vi "诊断标定3.vi"(8 "CAN端口":u16(ring), 9 "设备索引号":u16(ring), 10 "CAN卡类型":u32(ring)=21) -> ()   [LabVIEW 2013] (continued)
      n10 = property on="电池实际容量(A)" class="DigNum (严格)"("Disabled"=w43) -> ()  [unwired: 2 in, 2 out]
      n11 = property on="使用者" class="DigNum (严格)"("Disabled"=w43) -> ()  [unwired: 2 in, 2 out]
      n12 = property on="SOH(%)" class="DigNum (严格)"("Disabled"=w43) -> ()  [unwired: 2 in, 2 out]
      n13 = property on="电池额定容量(A)" class="DigNum (严格)"("Disabled"=w43) -> ()  [unwired: 2 in, 2 out]
      n14 = local write "主从选择"(enum32{"主板", "从板"}."主板" ("主从选择")) -> ()
      n15 = property on="SOC(%)" class="DigNum (严格)"("Disabled"=w43) -> ()  [unwired: 2 in, 2 out]
      n16 = local write "等级 2"(T19."从板信息" ("等级 2")) -> ()
      n17 = local write "主板2"(T8."项目信息" ("主从板")) -> ()
      n18 = property class="MCListbox (严格)"(reference=w48, "ItemNames"=w44) -> ()  [unwired: 1 in, 2 out]
      n19 = property class="MCListbox (严格)"(reference=w47, "ItemNames"=w44) -> ()  [unwired: 1 in, 2 out]
      n20 = property class="MCListbox (严格)"(reference=w46, "ItemNames"=w44) -> ()  [unwired: 1 in, 2 out]
      n21 = property class="Bool (严格)"(reference=w65, "BoolText.TextColor"=u32 87470) -> ()  [unwired: 1 in, 2 out]
      n22 = property class="Bool (严格)"(reference=w66, "BoolText.TextColor"=w40) -> ()  [unwired: 1 in, 2 out]
      n23 = local write "主从板"(enum32{"单选选项2", "单选选项1"}."单选选项1" ("主从板")) -> ()
      n24 = property on="项目信息2" class="Clust (严格)"("DisabledEnum"=w43) -> ()  [unwired: 2 in, 2 out]
      n25 = property on="系统时钟" class="Str"("Disabled"=w43) -> ()  [unwired: 2 in, 2 out]
      n26 = property on="配置文件版本" class="Str"("Disabled"=w43) -> ()  [unwired: 2 in, 2 out]
      n27 = property on="车架(牌)号" class="Str"("Disabled"=w43) -> ()  [unwired: 2 in, 2 out]
      n28 = property on="产品编号" class="Str"("Disabled"=w43) -> ()  [unwired: 2 in, 2 out]
      n29 = property on="从板号" class="DigNum (严格)"("NumText.BGColor"=w40) -> ()  [unwired: 2 in, 2 out]
      n30 = property on="单选选项2 2" class="Bool (严格)"("BoolText.TextColor"=w40) -> ()  [unwired: 2 in, 2 out]
      n31 = local write "面板选择"(T7."读写参数" ("面板选择")) -> ()
      n32 = property on="单选选项1" class="Bool (严格)"("BoolText.TextColor"=u32 5898201) -> ()  [unwired: 2 in, 2 out]
      n33 = property on="单选选项2" class="Bool (严格)"("BoolText.TextColor"=w40) -> ()  [unwired: 2 in, 2 out]
      n34 = local write "主界面选项"(enum32{"单选选项1", "单选选项2", "单选选项2 2", "单选选项2 3"}."单选选项1" ("主界面选项")) -> ()
      n35 = local write "判定3"(w50) -> ()
      n36 = local write "清BUFF"(w50) -> ()
      n37 = local write "1"(w50) -> ()
      n38 = property on="从板个数" class="DigNum (严格)"("Visible"=w50) -> ()  [unwired: 2 in, 2 out]
      n39 = property on="从板个数" class="DigNum (严格)"("NumText.BGColor"=u32 16448250) -> ()  [unwired: 2 in, 2 out]
      n40 = Not(x=w50) -> (.not. x?=w69:bool)
      n41 = local write "布尔"(w50) -> ()
      n42 = property on="主板选项" class="Tree (严格)"("Visible"=w50) -> ()  [unwired: 2 in, 2 out]
      n43 = property on="全部写入" class="Bool (严格)"("DisabledEnum"=2) -> ()  [unwired: 2 in, 2 out]
      n44 = property on="当前从板板号" class="DigNum (严格)"("Visible"=w69) -> ()  [unwired: 2 in, 2 out]
      n45 = property on="从板选项" class="Tree (严格)"("Visible"=w69) -> ()  [unwired: 2 in, 2 out]
      n46 = control-ref of="结果"() -> (w56:refnum<vi>)
      n47 = control-ref of="结果"() -> (w53:refnum<vi>)
      n48 = local write "强制停止版本读取"(w42) -> ()
      n49 = local write "强制终止读写标记"(w42) -> ()
      n50 = control-ref of="项目信息"() -> (w54:refnum<vi>)
      n51 = local write "判定2"(w42) -> ()
      n52 = local write "停止"(w42) -> ()
      n53 = local write "控制1"(w42) -> ()
      n54 = local write "消除"(w42) -> ()
      n55 = global write "EV05全局变量1.vi" "授权功能"(w42) -> ()
      n56 = local write "继电器超时处理"(w42) -> ()
      n57 = local write "1 6"(w42) -> ()
      n58 = local write "1 7"(w42) -> ()
      n59 = local write "1 8"(w42) -> ()
      n60 = local write "1 9"(w42) -> ()
      n61 = local write "1 10"(w42) -> ()
      n62 = local write "1 2"(w42) -> ()
      n63 = local write "1 3"(w42) -> ()
      n64 = local write "1 4"(w42) -> ()
      n65 = local write "1 5"(w42) -> ()
      n66 = local write "1 11"(w42) -> ()
      n67 = for {
        N: 100 -> [_]
        tunnel: w56 -> [w95]
        i -> [w93]
        n68 = Bundle(w93, 0) -> (w91:cluster{i32, i32})  [unwired: 1 out]
        n69 = property class="MCListbox (严格)"(reference=w95, "ActiveCell"=w91, "CellBG"=u32 16448250) -> ()  [unwired: 1 in, 2 out]
      }
      n70 = for {
        N: 100 -> [_]
        tunnel: w54 -> [w90]
        i -> [w89]
        n71 = Bundle(w89, 0) -> (w87:cluster{i32, i32})  [unwired: 1 out]
        n72 = property class="Tbl (严格)"(reference=w90, "Active Cell"=w87, "Cell BG Color"=u32 16448250) -> ()  [unwired: 1 in, 2 out]
      }
      n73 = for {
        N: 100 -> [_]
        tunnel: w53 -> [w100]
        i -> [w98]
        n74 = Bundle(w98, 0) -> (w96:cluster{i32, i32})  [unwired: 1 out]
        n75 = property class="MCListbox (严格)"(reference=w100, "ActiveCell"=w96, "CellBG"=u32 16448250) -> ()  [unwired: 1 in, 2 out]
      }
      n76 = stacked-sequence {
        tunnel: [_ w74] -> w49
        frame #0 {
          n77 = local read "设备索引号"() -> (w71:u16)
          n78 = local read "CAN卡类型"() -> (w70:u32)
          n79 = local read "CAN端口"() -> (w72:u16)
          n80 = dll-call lib="PTH1tabs FBluewave New EnergySVN_Work\nBNET01_BMStrunkBMS_Monitor_增加二维码data\nkerneldlls\nusbcan.dll" fn="VCI_ClearBuffer"("DeviceType"=w70, "DeviceInd"=w71, "CANInd"=w72) -> (error out=w73:errorcluster)  [unwired: 4 in, 4 out]
          n81 = call <vilib>:"Clear Errors.vi"("error in (no error)"=w73) -> ()  [unwired: 6 in, 1 out]
        }
        frame #1 {
          w81 = u8 0 items=["Normal", "Listen Only"] ("工作方式")
          w80 = u8 1 items=["Dual Filter", "Single Filter"] ("滤波方式")
          n82 = local read "设备索引号"() -> (w76:u16)
          n83 = local read "CAN卡类型"() -> (w75:u32)
          n84 = local read "CAN端口"() -> (w77:u16)
          n85 = call "CAN_Init-8.6.vi"("CAN卡类型"=w75, "设备索引号"=w76, "CAN端口"=w77, "操作类型"=enum16{"初始化CAN", "关闭CAN"}."初始化CAN", "滤波方式"=w80, "Accept Code"=u32 3221225472, "簇"=T21 {"打开CAN"=FALSE, "初始化CAN"=TRUE, "开始CAN"=TRUE, "重启"=FALSE, "关闭CAN"=FALSE}, "Mask Code"=u32 1073741823 ("Accept Code"), "工作方式"=w81, "是否滤波"=TRUE, "滤波选择"=T20 {"fiter_mode"=1, "fiter_endid"=402653184, "fiter_startid"=419430399}) -> ("error out"=w74:errorcluster)  [unwired: 3 in, 5 out]
        }
      }
      n86 = local write "加热继电器(从)"(w42) -> ()
      n87 = local write "风机继电器(从)"(w42) -> ()
      n88 = local write "DO1"(w42) -> ()
      n89 = local write "DO2"(w42) -> ()
      n90 = local write "DO1 2"(w42) -> ()
      n91 = local write "正级继电器"(w42) -> ()
      n92 = local write "负级继电器"(w42) -> ()
      n93 = local write "加热继电器"(w42) -> ()
      n94 = local write "充电继电器"(w42) -> ()
      n95 = local write "风机继电器"(w42) -> ()
      n96 = local write "预充电继电器"(w42) -> ()
      n97 = property on="保存版本信息" class="Bool (严格)"("Visible"=w42) -> ()  [unwired: 2 in, 2 out]
      n98 = property on="单个读取" class="Bool (严格)"("Visible"=w42) -> ()  [unwired: 2 in, 2 out]
      n99 = property on="单个写入" class="Bool (严格)"("Visible"=w42) -> ()  [unwired: 2 in, 2 out]
      n100 = local write "正级继电器 12"(w42) -> ()
      n101 = local write "正级继电器 2"(w42) -> ()
      n102 = local write "正级继电器 3"(w42) -> ()
      n103 = local write "正级继电器 4"(w42) -> ()
      n104 = local write "正级继电器 5"(w42) -> ()
      n105 = local write "正级继电器 6"(w42) -> ()
      n106 = local write "正级继电器 7"(w42) -> ()
      n107 = local write "正级继电器 8"(w42) -> ()
      n108 = local write "正级继电器 9"(w42) -> ()
      n109 = local write "正级继电器 10"(w42) -> ()
      n110 = local write "正级继电器 11"(w42) -> ()
      n111 = property on="从板号" class="DigNum (严格)"("Visible"=w42) -> ()  [unwired: 2 in, 2 out]
      "电池故障" <- w44
      "模块版本值" <- w61
      "硬件版本" <- w62
      "模块版本名称" <- w61
      "平台软件版本" <- w62
      "项目软件版本" <- w62
      "模块个数" <- u8[] [0, 0, 0, 0, 0, 0, 0, 0, 0, 0, 0, 0, 0, 0, 0, 0, 0, 0, 0, 0, 0, 0, 0, 0, 0, 0, 0, 0, 0, 0, 0, 0] ("模块个数")
    }
  }
  n112 = stacked-sequence {
    tunnel: [w101] -> w23
    frame #0 {
      n113 = call <vilib>:"Set Busy.vi"() -> ()  [unwired: 10 in, 2 out]
      n114 = disable-structure shown="禁用" {
        frame Disabled {
          n115 = control-ref of="主板选项"() -> (w220:refnum<vi>)
          n116 = stacked-sequence {
            tunnel: w220 -> [w222 w380 w418]
            frame #0 {
              # "加热和充电控制参数"
              n117 = global read "功能码全局.vi" "主板控制类信息10"() -> (w232:bool[])
              n118 = Index Array(array=w232) -> (element #5=w226:bool, element #6=w224:bool, element #7=w225:bool, element #8=w223:bool)  [unwired: 8 in, 4 out]
              n119 = Not Or(1:w225, 2:w226) -> (0:w231:bool)
              n120 = Not Or(1:w223, 2:w224) -> (0:w229:bool)
              n121 = for {
                N: 8 -> [_]
                tunnel: w222 -> [w352]
                tunnel: w231 -> [w348]
                tunnel: [w347] -> w230
                i -> [w350]
                n122 = Add(x=w350, y=69) -> (x+y=w351:i32)
                n123 = property class="Tree (严格)"(reference=w352, "Active Item Row Number"=w351, "Disabled?"=w348) -> (error out=w347:errorcluster)  [unwired: 1 in, 1 out]
              }
              n124 = for {
                N: 9 -> [_]
                tunnel: w222 -> [w346]
                tunnel: w229 -> [w342]
                tunnel: w230 -> [w341]
                tunnel: [w340] -> w221
                i -> [w344]
                n125 = Add(x=w344, y=77) -> (x+y=w345:i32)
                n126 = property class="Tree (严格)"(reference=w346, error in=w341, "Active Item Row Number"=w345, "Disabled?"=w342) -> (error out=w340:errorcluster)  [unwired: 1 out]
              }
              n127 = stacked-sequence {
                tunnel: w222 -> [w252 _ _]
                tunnel: w221 -> [w251 _ _]
                frame #0 {
                  # "电池信息"
                  n128 = global read "功能码全局.vi" "主板版本号11"() -> (w253:bool[])
                  n129 = global read "功能码全局.vi" "主板项目信息4"() -> (w235:bool[])
                  n130 = Index Array(array=w253) -> (element #1=w249:bool, element #2=w248:bool, element #3=w242:bool, element #4=w236:bool, element #6=w241:bool, element #7=w240:bool, element #8=w239:bool)  [unwired: 8 in, 1 out]
                  n131 = Index Array(array=w235, index=4 ("索引")) -> (element=w233:bool)
                  n132 = Or(x=w242, y=w236) -> (x .or. y?=w237:bool)
                  n133 = Not(x=w240) -> (.not. x?=w244:bool)
                  n134 = Not(x=w239) -> (.not. x?=w243:bool)
                  n135 = Not(x=w241) -> (.not. x?=w245:bool)
                  n136 = property on="硬件版本号" class="Str"("Visible"=w242) -> ()  [unwired: 2 in, 2 out]
                  n137 = property on="读硬件版本号" class="Bool (严格)"("Visible"=w242) -> ()  [unwired: 2 in, 2 out]
                  n138 = property on="项目软件版本号" class="Str"("Visible"=w242) -> ()  [unwired: 2 in, 2 out]
                  n139 = property on="项目软本读取" class="Bool (严格)"("Visible"=w242) -> ()  [unwired: 2 in, 2 out]
                  n140 = property on="继电器屏1 2" class="TabCtl (严格)"("Visible"=w245) -> ()  [unwired: 2 in, 2 out]
                  n141 = property on="均衡屏" class="TabCtl (严格)"("Visible"=w243) -> ()  [unwired: 2 in, 2 out]
                  n142 = property on="继电器屏1 2" class="TabCtl (严格)"("Visible"=w245) -> ()  [unwired: 2 in, 2 out]
                  n143 = property on="DO屏" class="TabCtl (严格)"("Visible"=w244) -> ()  [unwired: 2 in, 2 out]
                  n144 = Compound Arithmetic op=OR(w241, w240, w239) -> (w238:bool)
                  n145 = Not Or(1:w248, 2:w249) -> (0:w247:bool)
                  n146 = stacked-sequence {
                    tunnel: w238 -> [_ w258 _]
                    tunnel: w237 -> [_ _ w262]
                    tunnel: w233 -> [w254 _ _]
                    frame #0 {
                      n147 = case shown="真" w254 {
                        frame False {
                        }
                        frame True {
                          n148 = local write "主界面选项"(enum32{"单选选项1", "单选选项2", "单选选项2 2", "单选选项2 3"}."单选选项2 3" ("主界面选项")) -> ()
                          n149 = local write "面板选择"(T7."高压板校正" ("面板选择")) -> ()
                        }
                      }
                      n150 = control-ref of="单选选项2 3"() -> (w255:refnum<vi>)
                      n151 = property class="Bool (严格)"(reference=w255, "Visible"=w254) -> ()  [unwired: 1 in, 2 out]
                    }
                    frame #1 {
                      n152 = control-ref of="单选选项2 2"() -> (w259:refnum<vi>)
                      n153 = case shown="真" w258 {
                        frame False {
                        }
                        frame True {
                          n154 = local write "主界面选项"(enum32{"单选选项1", "单选选项2", "单选选项2 2", "单选选项2 3"}."单选选项2 2" ("主界面选项")) -> ()
                          n155 = local write "面板选择"(enum32{"读写参数", "版本读取", "其它诊断"}."其它诊断" ("选项卡控件 2")) -> ()
                        }
                      }
                      n156 = property class="Bool (严格)"(reference=w259, "Visible"=w258) -> ()  [unwired: 1 in, 2 out]
                    }
                    frame #2 {
                      n157 = control-ref of="单选选项2"() -> (w263:refnum<vi>)
                      n158 = case shown="真" w262 {
                        frame False {
                        }
                        frame True {
                          n159 = local write "主界面选项"(enum32{"单选选项1", "单选选项2", "单选选项2 2", "单选选项2 3"}."单选选项2" ("主界面选项")) -> ()
                          n160 = local write "面板选择"(enum32{"读写参数", "版本读取", "其它诊断"}."版本读取" ("选项卡控件 2")) -> ()
                        }
                      }
                      n161 = property class="Bool (严格)"(reference=w263, "Visible"=w262) -> ()  [unwired: 1 in, 2 out]
                    }
                  }
                  n162 = for {
                    N: 5 -> [_]
                    tunnel: w252 -> [w272]
                    tunnel: w247 -> [w268]
                    tunnel: w251 -> [w267]
                    tunnel: [w266] -> w250
                    i -> [w270]
                    n163 = Add(x=w270, y=86) -> (x+y=w271:i32)
                    n164 = property class="Tree (严格)"(reference=w272, error in=w267, "Active Item Row Number"=w271, "Disabled?"=w268) -> (error out=w266:errorcluster)  [unwired: 1 out]
                  }
                  n165 = property on="模块软件版本 2" class="MCListbox (严格)"("Visible"=w236) -> ()  [unwired: 2 in, 2 out]
                  n166 = property on="模块软件版本" class="Enum (严格)"("Visible"=w236) -> ()  [unwired: 2 in, 2 out]
                  n167 = property on="平台软件版本号" class="Str"("Visible"=w236) -> ()  [unwired: 2 in, 2 out]
                  n168 = property on="模块版本读取" class="Bool (严格)"("Visible"=w236) -> ()  [unwired: 2 in, 2 out]
                  n169 = property on="平台软件版本读取" class="Bool (严格)"("Visible"=w236) -> ()  [unwired: 2 in, 2 out]
                  n170 = call <vilib>:"Clear Errors.vi"("error in (no error)"=w250) -> ()  [unwired: 6 in, 1 out]
                }
                frame #1 {
                  n171 = global read "功能码全局.vi" "主板项目信息7"() -> (w312:bool[])
                  n172 = global read "功能码全局.vi" "主板控制类信息10"() -> (w308:bool[])
                  n173 = global read "功能码全局.vi" "主板故障阀值9"() -> (w311:bool[])
                  n174 = global read "功能码全局.vi" "主板项目信息4"() -> (w290:bool[])
                  n175 = global read "功能码全局.vi" "主板项目信息5"() -> (w299:bool[])
                  n176 = global read "功能码全局.vi" "主板项目信息6"() -> (w289:bool[])
                  n177 = global read "功能码全局.vi" "主板版本号11"() -> (w298:bool[])
                  n178 = Delete From Array(array=w289, length=1 ("长度"), index=0 ("索引")) -> (deleted portion=w300:bool[], array with subset deleted=w316:bool[])
                  n179 = Index Array(array=w290, index #1=5 ("索引"), index #2=6 ("索引"), index #3=7 ("索引")) -> (element #1=w301:bool, element #2=w317:bool, element #3=w273:bool)
                  n180 = Index Array(array=w298) -> (element #1=w305:bool, element #2=w321:bool)  [unwired: 2 in]
                  n181 = Array Subset(array=w311, index=2 ("索引"), length=3 ("长度")) -> (w303:bool[])
                  n182 = Delete From Array(array=w312, length=3 ("索引"), index=2 ("长度")) -> (deleted portion=w302:bool[], array with subset deleted=w318:bool[])
                  n183 = Array Subset(array=w308, index=4 ("索引"), length=2 ("长度")) -> (w304:bool[])
                  n184 = global read "功能码全局.vi" "18"() -> (w281:bool[])
                  n185 = global read "功能码全局.vi" "16"() -> (w282:bool[])
                  n186 = Insert Into Array(array=w299, new element #1=w300, new element #2=w301, new element #3=w302, new element #4=w303, new element #5=w304, new element #6=w305) -> (w322:bool[])  [unwired: 1 in]
                  n187 = Array Subset(array=w308, index=6 ("索引"), length=2 ("长度")) -> (w320:bool[])
                  n188 = Array Subset(array=w311, index=5 ("索引"), length=3 ("长度")) -> (w319:bool[])
                  n189 = And Array Elements(Boolean array=w322) -> (logical AND=w287:bool)
                  n190 = Array Subset(array=w281, index=0 ("索引"), length=8 ("长度")) -> (w279:bool[])
                  n191 = Array Subset(array=w282, index=4 ("索引"), length=4 ("长度")) -> (w278:bool[])
                  n192 = Or Array Elements(Boolean array=w322) -> (logical OR=w274:bool)
                  n193 = Insert Into Array(array=w316, new element #1=w317, new element #2=w318, new element #3=w319, new element #4=w320, new element #5=w321) -> (w323:bool[])  [unwired: 1 in]
                  n194 = property on="全部读取" class="Bool (严格)"("Visible"=w287) -> ()  [unwired: 2 in, 2 out]
                  n195 = global read "功能码全局.vi" "15"() -> (w280:bool[])
                  n196 = And Array Elements(Boolean array=w323) -> (logical AND=w288:bool)
                  n197 = property on="全部写入" class="Bool (严格)"("Visible"=w288) -> ()  [unwired: 2 in, 2 out]
                  n198 = Or Array Elements(Boolean array=w323) -> (logical OR=w324:bool)
                  n199 = Insert Into Array(array=w280, new element #1=w279, new element #2=w278) -> (w277:bool[])  [unwired: 1 in]
                  n200 = Or Array Elements(Boolean array=w277) -> (logical OR=w276:bool)
                  n201 = Compound Arithmetic op=OR(w273, w274, w324, w276) -> (w325:bool)
                  n202 = case shown="真" w325 {
                    frame False {
                    }
                    frame True {
                      n203 = local write "主界面选项"(enum32{"单选选项1", "单选选项2", "单选选项2 2", "单选选项2 3"}."单选选项1" ("主界面选项")) -> ()
                      n204 = local write "面板选择"(enum32{"读写参数", "版本读取", "其它诊断"}."读写参数" ("选项卡控件 2")) -> ()
                    }
                  }
                  n205 = property on="单选选项1" class="Bool (严格)"("Visible"=w325) -> ()  [unwired: 2 in, 2 out]
                }
                frame #2 {
                  n206 = control-ref of="单选选项2 2"() -> (w332:refnum<vi>)
                  n207 = control-ref of="单选选项2 3"() -> (w328:refnum<vi>)
                  n208 = control-ref of="单选选项2"() -> (w334:refnum<vi>)
                  n209 = control-ref of="单选选项1"() -> (w333:refnum<vi>)
                  n210 = local read "主界面选项"() -> (w337:enum32{"单选选项1", "单选选项2", "单选选项2 2", "单选选项2 3"})
                  n211 = Build Array(w333, w334, w332, w328) -> (w331:refnum<vi>[])
                  n212 = Delete From Array(array=w331, index=w337) -> (deleted portion=w335:refnum<vi>, array with subset deleted=w336:refnum<vi>[])  [unwired: 1 in]
                  n213 = property class="Bool (严格)"(reference=w335, "BoolText.TextColor"=u32 87470) -> ()  [unwired: 1 in, 2 out]
                  n214 = for {
                    tunnel: u32 16777215 -> [w339]
                    tunnel: w336 -> [w338] mode=indexing
                    n215 = property class="Bool (严格)"(reference=w338, "BoolText.TextColor"=w339) -> ()  [unwired: 1 in, 2 out]
                  }
                }
              }
            }
            frame #1 {
              # "项目信息"
              # "SOC"
              # "SOH"
              # "电池额定实际容量"
              # "车牌号"
              # "产品编号"
              # "电压个数"
              # "通道电压数"
              # "温度个数"
              # "电压起始值"
              # "温度起始值"
              # "配置文件版本"
              # "系统时钟"
              # "校正时钟"
              n216 = global read "功能码全局.vi" "主板项目信息5"() -> (w413:bool[])
              n217 = global read "功能码全局.vi" "主板项目信息6"() -> (w412:bool[])
              n218 = global read "功能码全局.vi" "主板项目信息7"() -> (w389:bool[])
              n219 = global read "功能码全局.vi" "主板项目信息4"() -> (w360:bool[])
              n220 = Index Array(array=w413) -> (element #1=w410:bool, element #2=w407:bool, element #3=w404:bool, element #4=w401:bool, element #5=w397:bool, element #6=w395:bool, element #7=w392:bool, element #8=w388:bool)  [unwired: 8 in]
              n221 = Index Array(array=w412) -> (element #1=w385:bool, element #2=w409:bool, element #3=w406:bool, element #4=w403:bool, element #5=w400:bool, element #6=w396:bool, element #7=w394:bool, element #8=w391:bool)  [unwired: 8 in]
              n222 = Index Array(array=w389) -> (element #1=w387:bool, element #2=w384:bool, element #3=w382:bool, element #4=w377:bool, element #5=w374:bool, element #6=w381:bool, element #7=w375:bool, element #8=w373:bool)  [unwired: 8 in]
              n223 = Index Array(array=w360) -> (element #6=w356:bool, element #7=w355:bool, element #8=w359:bool)  [unwired: 8 in, 5 out]
              n224 = Not(x=w359) -> (.not. x?=w358:bool)
              n225 = Not Or(1:w355, 2:w356) -> (0:w354:bool)
              n226 = Not Or(1:w409, 2:w410) -> (0:w372:bool)
              n227 = Not Or(1:w406, 2:w407) -> (0:w371:bool)
              n228 = Not Or(1:w403, 2:w404) -> (0:w370:bool)
              n229 = Not Or(1:w400, 2:w401) -> (0:w369:bool)
              n230 = Not Or(1:w396, 2:w397) -> (0:w368:bool)
              n231 = Not Or(1:w394, 2:w395) -> (0:w367:bool)
              n232 = Not Or(1:w391, 2:w392) -> (0:w366:bool)
              n233 = Not Or(1:w387, 2:w388) -> (0:w365:bool)
              n234 = Not Or(1:w381, 2:w382) -> (0:w363:bool)
              n235 = Not Or(1:w373, 2:w374) -> (0:w361:bool)
              n236 = Not Or(1:w375, 2:w377) -> (0:w362:bool)
              n237 = Not Or(1:w384, 2:w385) -> (0:w364:bool)
              n238 = Compound Arithmetic op=OR(w358, w372, w371, w370, w369, w368, w367, w366, w365, w364, w363, w362, w361) -> (w353:bool)
              "项目信息结果" <- w353
              n239 = property class="Tree (严格)"(reference=w380, "Active Item Row Number"=9 ("活动项:行数"), "Disabled?"=w354, "Active Item Row Number"=1 ("活动项:行数"), "Disabled?"=w353, "Active Item Row Number"=0 ("活动项:行数"), "Disabled?"=w358, "Active Item Row Number"=3 ("活动项:行数"), "Disabled?"=w372, "Active Item Row Number"=4 ("活动项:行数"), "Disabled?"=w371, "Active Item Row Number"=5 ("活动项:行数"), "Disabled?"=w370, "Active Item Row Number"=6 ("活动项:行数"), "Disabled?"=w369, "Active Item Row Number"=7 ("活动项:行数"), "Disabled?"=w368, "Active Item Row Number"=8 ("活动项:行数"), "Disabled?"=w367, "Active Item Row Number"=11 ("活动项:行数"), "Disabled?"=w366, "Active Item Row Number"=12 ("活动项:行数"), "Disabled?"=w365, "Active Item Row Number"=13 ("活动项:行数"), "Disabled?"=w364, "Active Item Row Number"=2 ("活动项:行数"), "Disabled?"=w363, "Active Item Row Number"=10 ("活动项:行数"), "Disabled?"=w362, "Active Item Row Number"=14 ("活动项:行数"), "Disabled?"=w361) -> ()  [unwired: 1 in, 2 out]
            }
            frame #2 {
              w423 = 18
              # "一二三级故障"
              n240 = global read "功能码全局.vi" "主板故障阀值9"() -> (w429:bool[])
              n241 = Index Array(array=w429) -> (element #3=w428:bool, element #4=w425:bool, element #5=w422:bool, element #6=w427:bool, element #7=w424:bool, element #8=w421:bool)  [unwired: 8 in, 2 out]
              n242 = Not Or(1:w427, 2:w428) -> (0:w417:bool)
              n243 = Not Or(1:w424, 2:w425) -> (0:w415:bool)
              n244 = Not Or(1:w421, 2:w422) -> (0:w416:bool)
              n245 = for {
                N: w423 -> [_]
                tunnel: w418 -> [w449]
                tunnel: w417 -> [w445]
                tunnel: [w444] -> w426
                i -> [w447]
                n246 = Add(x=w447, y=15) -> (x+y=w448:i32)
                n247 = property class="Tree (严格)"(reference=w449, "Active Item Row Number"=w448, "Disabled?"=w445) -> (error out=w444:errorcluster)  [unwired: 1 in, 1 out]
              }
              n248 = for {
                N: w423 -> [_]
                tunnel: w418 -> [w443]
                tunnel: w415 -> [w439]
                tunnel: w426 -> [w438]
                tunnel: [w437] -> w420
                i -> [w441]
                n249 = Add(x=w441, y=33) -> (x+y=w442:i32)
                n250 = property class="Tree (严格)"(reference=w443, error in=w438, "Active Item Row Number"=w442, "Disabled?"=w439) -> (error out=w437:errorcluster)  [unwired: 1 out]
              }
              n251 = for {
                N: w423 -> [_]
                tunnel: w418 -> [w436]
                tunnel: w416 -> [w432]
                tunnel: w420 -> [w431]
                tunnel: [w430] -> w419
                i -> [w434]
                n252 = Add(x=w434, y=51) -> (x+y=w435:i32)
                n253 = property class="Tree (严格)"(reference=w436, error in=w431, "Active Item Row Number"=w435, "Disabled?"=w432) -> (error out=w430:errorcluster)  [unwired: 1 out]
              }
              n254 = call <vilib>:"Clear Errors.vi"("error in (no error)"=w419) -> ()  [unwired: 6 in, 1 out]
            }
          }
        }
        frame Enabled {
        }
      }
      n255 = disable-structure shown="禁用" {
        disable-tunnel: [w102 _] -> w101
        frame Disabled {
          n256 = control-ref of="从板选项"() -> (w103:refnum<vi>)
          n257 = stacked-sequence {
            tunnel: w103 -> [w106 w143 w185]
            tunnel: [w104 _ _] -> w102
            frame #0 {
              n258 = global read "功能码全局.vi" "15"() -> (w129:bool[])
              n259 = global read "功能码全局.vi" "16"() -> (w120:bool[])
              n260 = Index Array(array=w129) -> (element #1=w128:bool, element #2=w126:bool, element #3=w124:bool, element #4=w122:bool, element #5=w127:bool, element #6=w125:bool, element #7=w123:bool, element #8=w121:bool)  [unwired: 8 in]
              n261 = Index Array(array=w120) -> (element #5=w111:bool, element #6=w119:bool, element #7=w110:bool, element #8=w118:bool)  [unwired: 8 in, 4 out]
              n262 = Not Or(1:w118, 2:w119) -> (0:w108:bool)
              n263 = Not Or(1:w110, 2:w111) -> (0:w109:bool)
              n264 = Not Or(1:w127, 2:w128) -> (0:w114:bool)
              n265 = Not Or(1:w125, 2:w126) -> (0:w115:bool)
              n266 = Not Or(1:w123, 2:w124) -> (0:w116:bool)
              n267 = Not Or(1:w121, 2:w122) -> (0:w117:bool)
              n268 = Compound Arithmetic op=OR(w114, w115, w116, w117, w108) -> (w113:bool)
              "从板项目信息" <- w113
              n269 = property class="Tree (严格)"(reference=w106, "Active Item Row Number"=1 ("活动项:行数"), "Disabled?"=w113, "Active Item Row Number"=2 ("活动项:行数"), "Disabled?"=w114, "Active Item Row Number"=3 ("活动项:行数"), "Disabled?"=w115, "Active Item Row Number"=4 ("活动项:行数"), "Disabled?"=w116, "Active Item Row Number"=5 ("活动项:行数"), "Disabled?"=w117, "Active Item Row Number"=0 ("活动项:行数"), "Disabled?"=w109) -> (error out=w105:errorcluster)  [unwired: 1 in, 1 out]
              n270 = for {
                N: 8 -> [_]
                tunnel: w106 -> [w141]
                tunnel: w108 -> [w137]
                tunnel: w105 -> [w136]
                tunnel: [w135] -> w104
                i -> [w139]
                n271 = Add(x=w139, y=6) -> (x+y=w140:i32)
                n272 = property class="Tree (严格)"(reference=w141, error in=w136, "Active Item Row Number"=w140, "Disabled?"=w137) -> (error out=w135:errorcluster)  [unwired: 1 out]
              }
              n273 = call <vilib>:"Clear Errors.vi"("error in (no error)"=w104) -> ()  [unwired: 6 in, 1 out]
            }
            frame #1 {
              w154 = 8
              n274 = global read "功能码全局.vi" "18"() -> (w163:bool[])
              n275 = Index Array(array=w163) -> (element #1=w146:bool, element #2=w147:bool, element #3=w162:bool, element #4=w157:bool, element #5=w151:bool, element #6=w161:bool, element #7=w156:bool, element #8=w150:bool)  [unwired: 8 in]
              n276 = Not Or(1:w147, 2:w146) -> (0:w142:bool)
              n277 = property class="Tree (严格)"(reference=w143, "Active Item Row Number"=46 ("活动项:行数"), "Disabled?"=w142, "Active Item Row Number"=47 ("活动项:行数"), "Disabled?"=w142, "Active Item Row Number"=48 ("活动项:行数"), "Disabled?"=w142) -> ()  [unwired: 1 in, 2 out]
              n278 = Not Or(1:w150, 2:w151) -> (0:w149:bool)
              n279 = Not Or(1:w161, 2:w162) -> (0:w160:bool)
              n280 = Not Or(1:w156, 2:w157) -> (0:w155:bool)
              n281 = for {
                N: w154 -> [_]
                tunnel: w143 -> [w184]
                tunnel: w160 -> [w180]
                tunnel: "error out" -> [w179]
                tunnel: [w178] -> w158
                i -> [w182]
                n282 = Add(x=w182, y=14) -> (x+y=w183:i32)
                n283 = property class="Tree (严格)"(reference=w184, error in=w179, "Active Item Row Number"=w183, "Disabled?"=w180) -> (error out=w178:errorcluster)  [unwired: 1 out]
              }
              n284 = for {
                N: w154 -> [_]
                tunnel: w143 -> [w177]
                tunnel: w155 -> [w173]
                tunnel: w158 -> [w172]
                tunnel: [w171] -> w153
                i -> [w175]
                n285 = Add(x=w175, y=22) -> (x+y=w176:i32)
                n286 = property class="Tree (严格)"(reference=w177, error in=w172, "Active Item Row Number"=w176, "Disabled?"=w173) -> (error out=w171:errorcluster)  [unwired: 1 out]
              }
              n287 = for {
                N: w154 -> [_]
                tunnel: w143 -> [w170]
                tunnel: w149 -> [w166]
                tunnel: w153 -> [w165]
                tunnel: [w164] -> w152
                i -> [w168]
                n288 = Add(x=w168, y=30) -> (x+y=w169:i32)
                n289 = property class="Tree (严格)"(reference=w170, error in=w165, "Active Item Row Number"=w169, "Disabled?"=w166) -> (error out=w164:errorcluster)  [unwired: 1 out]
              }
              n290 = call <vilib>:"Clear Errors.vi"("error in (no error)"=w152) -> ()  [unwired: 6 in, 1 out]
            }
            frame #2 {
              n291 = global read "功能码全局.vi" "23"() -> (w209:bool[])
              n292 = global read "功能码全局.vi" "24"() -> (w207:bool[])
              n293 = Index Array(array=w209) -> (element #3=w208:bool, element #4=w205:bool, element #5=w203:bool, element #6=w201:bool, element #7=w199:bool, element #8=w197:bool)  [unwired: 8 in, 2 out]
              n294 = Index Array(array=w207) -> (element #3=w206:bool, element #4=w204:bool, element #5=w202:bool, element #6=w200:bool, element #7=w198:bool, element #8=w196:bool)  [unwired: 8 in, 2 out]
              n295 = Not Or(1:w206, 2:w208) -> (0:w195:bool)
              n296 = Not Or(1:w204, 2:w205) -> (0:w190:bool)
              n297 = Not Or(1:w202, 2:w203) -> (0:w191:bool)
              n298 = Not Or(1:w200, 2:w201) -> (0:w192:bool)
              n299 = Not Or(1:w198, 2:w199) -> (0:w194:bool)
              n300 = Not Or(1:w196, 2:w197) -> (0:w193:bool)
              n301 = Build Array(w195, w195, w194, w193, w192, w191, w190) -> (w188:bool[])
              n302 = And Array Elements(Boolean array=w188) -> (logical AND=w189:bool)
              n303 = Insert Into Array(array=w188, index=0 ("索引"), new element=w189) -> (w186:bool[])
              n304 = for {
                N: 8 -> [_]
                tunnel: w185 -> [w219]
                tunnel: w186 -> [w215] mode=indexing
                tunnel: errorcluster {"status"=FALSE, "code"=0, "source"=""} ("error out 2") -> [w214]
                tunnel: [w213] -> w211
                i -> [w217]
                n305 = Add(x=w217, y=38) -> (x+y=w218:i32)
                n306 = property class="Tree (严格)"(reference=w219, error in=w214, "Active Item Row Number"=w218, "Disabled?"=w215) -> (error out=w213:errorcluster)  [unwired: 1 out]
              }
              n307 = call <vilib>:"Clear Errors.vi"("error in (no error)"=w211) -> ()  [unwired: 6 in, 1 out]
            }
          }
        }
        frame Enabled {
        }
      }
    }
  }
  n308 = local write "项目信息 2"(string[][] [["电压个数", "36"], ["温度个数", "45"], ["第一个保险通道", "0"], ["第一个保险位置", "0"], ["第二个保险通道", "0"], ["第二个保险位置", "0"], ["第三个保险通道", "0"], ["第三个保险位置", "0"], ["第四个保险通道", "0"], ["第四个保险位置", "0"], ["第五个保险通道", "0"], ["第五个保险位置", "0"], ["第六个保险通道", "0"], ["第六个保险位置", "0"], ["第七个保险通道", "0"], ["第七个保险位置", "0"], ["第八个保险通道", "0"], ["第八个保险位置", "0"], ["第九个保险通道", "0"], ["第九个保险位置", "0"], ["第十个保险通道", "0"], ["第十个保险位置", "0"], ["第1通道电压个数", "11"], ["第2通道电压个数", "12"], ["第3通道电压个数", "12"], ["第4通道电压个数", "12"], ["第5通道电压个数", "12"]] ("项目信息 2")) -> ()
  n309 = Index Array(array=w13, index (col)=0 ("索引 (行)")) -> (element=w16:string[])  [unwired: 1 in]
  n310 = Index Array(array=w13, index (col)=1 ("禁用的索引 (列)")) -> (element=w6:string[])  [unwired: 1 in]
  n311 = local read "从板个数"() -> (w8:dbl)
  n312 = Array Subset(array=w16, index=0 ("索引"), length=w8) -> (w15:string[])
  n313 = Array Subset(array=w16, index=10 ("索引"), length=w8) -> (w14:string[])
  n314 = Array Subset(array=w6, index=0 ("索引"), length=w8) -> (w12:string[])
  n315 = Array Subset(array=w6, index=10 ("索引"), length=w8) -> (w7:string[])
  n316 = Insert Into Array(array=w15, new element=w14) -> (w5:string[])  [unwired: 1 in]
  n317 = Insert Into Array(array=w12, new element=w7) -> (w4:string[])  [unwired: 1 in]
  n318 = stacked-sequence {
    tunnel: w20 -> [_]
    tunnel: w23 -> [_]
    frame #0 {
      n319 = call <vilib>:"Unset Busy.vi"() -> ()  [unwired: 11 in, 1 out]
    }
  }
  n320 = Build Array(w5, w4) -> (w3:string[][])
  n321 = local write "停止"(FALSE ("停止")) -> ()
  n322 = Transpose 2D Array(2D array=w3) -> (transposed array=w2:string[][])
  n323 = Obtain Queue(name (unnamed)=w37, element data type=w37, error in (no error)=w20) -> (queue out=w36:refnum<queue>, error out=w35:errorcluster)  [unwired: 2 in, 1 out]
  n324 = local write "项目信息"(w2) -> ()
  n325 = Obtain Queue(element data type="读参数") -> (queue out=w25:refnum<queue>, error out=w24:errorcluster)  [unwired: 4 in, 1 out]
  n326 = while {
    tunnel: w25 -> [w461]
    tunnel: w24 -> [w460]
    tunnel: [w459] -> w28
    tunnel: [w458] -> w27
    tunnel: w20 -> [_]
    tunnel: w23 -> [w450]
    stop <- w457 stop-if-true
    n327 = local read "停止"() -> (w457:bool)
    n328 = local read "设备索引号"() -> (w454:u16)
    n329 = local read "CAN卡类型"() -> (w455:u32)
    n330 = local read "CAN端口"() -> (w453:u16)
    n331 = call "receiver-8.6.vi"("错误输入（无错误）"=w450, "CAN端口"=w453, "设备索引号"=w454, "CAN卡类型"=w455) -> ("错误输出"=w456:errorcluster, "输出簇"=w452:T22, "接收成功"=w451:bool)  [unwired: 3 out]
    n332 = call <vilib>:"Clear Errors.vi"("error in (no error)"=w456) -> ()  [unwired: 6 in, 1 out]
    n333 = case shown="真" w451 {
      tunnel: w460 -> [w462 w468]
      tunnel: w452 -> [_ w467]
      tunnel: w461 -> [w463 w466]
      tunnel: [w463 w465] -> w459
      tunnel: [w462 w464] -> w458
      frame False {
      }
      frame True {
        n334 = Enqueue Element(queue=w466, element=w467, error in (no error)=w468) -> (queue out=w465:refnum<queue>, error out=w464:errorcluster)  [unwired: 2 out]
      }
    }
  }
  n335 = while {
    tunnel: w25 -> [w476]
    tunnel: w24 -> [w475]
    stop <- w469 stop-if-true
    n336 = local read "停止"() -> (w469:bool)
    n337 = local read "控制1"() -> (w471:bool)
    n338 = Dequeue Element(queue=w476, timeout in ms (-1)=200 ("超时毫秒(-1)"), error in (no error)=w475) -> (element=w474:T3, error out=w473:errorcluster)  [unwired: 2 out]
    n339 = case shown="无错误" w473 {
      tunnel: w474 -> [w481 _]
      tunnel: "写?" -> [w478 _]
      tunnel: w471 -> [w477 _]
      frame No Error {
        n340 = Unbundle(w481) -> ("return type"=w480:u32, "pReceive"=w479:T23)
        n341 = for {
          N: w480 -> [_]
          tunnel: w479 -> [w485] mode=indexing
          tunnel: w478 -> [w483]
          tunnel: w477 -> [w482]
          n342 = Unbundle By Name(w485) -> ("ID"=w486:u32)
          n343 = call "ID解析.vi"("ID"=w486) -> ("PDU(1)"=w484:i32)  [unwired: 10 out]
          n344 = case shown="18" w484 {
            tunnel: w485 -> [_ w496]
            tunnel: w483 -> [_ w488]
            tunnel: w482 -> [_ w487]
            frame 0, Default {
            }
            frame 24 {
              n345 = local read "主从选择"() -> (w489:enum32{"主板", "从板"})
              n346 = local read "设备索引号"() -> (w492:u16)
              n347 = local read "CAN卡类型"() -> (w491:u32)
              n348 = local read "CAN端口"() -> (w493:u16)
              n349 = disable-structure shown="禁用" {
                disable-tunnel: w496 -> [w499 _]
                frame Disabled {
                  n350 = call "标定授权读取.vi"("VCI_Receive"=w499) -> ()  [unwired: 1 out]
                }
                frame Enabled {
                }
              }
              n351 = case shown="\"从板\"" w489 {
                tunnel: [0 ("FUNC") w498] -> w490
                frame "主板", Default {
                }
                frame "从板" {
                  n352 = local read "从板号"() -> (w498:u8)
                }
              }
              n353 = local read "面板选择"() -> (w495:T7)
              n354 = case shown="\"读写参数\", 默认" w495 {
                tunnel: w488 -> [w504 _ _ _]
                tunnel: "命令" -> [w505 w608 w863 w1003]
                tunnel: w489 -> [w514 _ w871 w1011]
                tunnel: w496 -> [_ _ _ _]
                tunnel: w496 -> [w510 w609 w865 w1005]
                tunnel: w493 -> [w509 w610 w866 w1006]
                tunnel: w492 -> [w508 w611 w867 w1007]
                tunnel: w491 -> [w507 w612 w868 w1008]
                tunnel: w490 -> [w506 _ w864 w1004]
                tunnel: w487 -> [w500 _ _ _]
                frame "读写参数", Default {
                  n355 = local read "命令序号"() -> (w503:u8)
                  n356 = call "多帧接收机制(EV05).vi"("can卡类型"=w507, "设备索引号"=w508, "CAN端口"=w509, "VCI_Receive"=w510, "命令"=w505, "板号"=w506, "写?"=w504, "命令序号"=w503) -> ("错误信号"=w501:bool, "错误代码"=w513:i32, "输出数组"=w512:u8[], "读错误代码"=w502:u8[], "结束信号"=w511:bool)  [unwired: 7 out]
                  n357 = case shown="假" w504 {
                    tunnel: w511 -> [w524 w591]
                    tunnel: w513 -> [w523 w590]
                    tunnel: w503 -> [w522 _]
                    tunnel: w512 -> [w521 _]
                    tunnel: w505 -> [w520 _]
                    tunnel: w514 -> [w518 w589]
                    tunnel: w502 -> [w517 _]
                    tunnel: w501 -> [w516 _]
                    tunnel: w500 -> [w515 _]
                    frame False {
                      # "读参数"
                      n358 = And(x=w515, y=w524) -> (x .and. y?=w519:bool)
                      n359 = case shown="真" w519 {
                        tunnel: w523 -> [_ w535]
                        tunnel: w522 -> [_ w534]
                        tunnel: w521 -> [_ w533]
                        tunnel: w520 -> [_ w532]
                        tunnel: w518 -> [_ w528]
                        tunnel: w517 -> [_ w526]
                        tunnel: w516 -> [_ w527]
                        frame False {
                        }
                        frame True {
                          n360 = case shown="假" w527 {
                            tunnel: w535 -> [w546 _]
                            tunnel: w534 -> [w545 _]
                            tunnel: w533 -> [w544 _]
                            tunnel: w532 -> [w542 _]
                            tunnel: w528 -> [w538 _]
                            tunnel: w526 -> [_ w574]
                            frame False {
                              n361 = case shown="\"主板\", 默认" w538 {
                                tunnel: [w548 _] -> w541
                                tunnel: [_ w562] -> w540
                                tunnel: [w547 _] -> w537
                                frame "主板", Default {
                                n362 = stacked-sequence {
                                tunnel: [_ w561] -> w548
                                tunnel: [w549 _] -> w547
                                frame #0 {
                                n363 = control-ref of="一级故障"() -> (w555:refnum<vi>)
                                n364 = control-ref of="一级故障 2"() -> (w557:refnum<vi>)
                                n365 = control-ref of="一级故障 3"() -> (w558:refnum<vi>)
                                n366 = control-ref of="加热控制参数"() -> (w559:refnum<vi>)
                                n367 = control-ref of="充电控制参数"() -> (w560:refnum<vi>)
                                n368 = control-ref of="电池信息"() -> (w553:refnum<vi>)
                                n369 = control-ref of="项目信息"() -> (w556:refnum<vi>)
                                n370 = control-ref of="项目信息2"() -> (w554:refnum<vi>)
                                n371 = control-ref of="高压参数"() -> (w552:refnum<vi>)
                                n372 = local read "主板数据"() -> (w551:T4)
                                n373 = Bundle(cluster=w551, "项目信息"=w556, "一级故障 4"=w554, "一级故障"=w555, "一级故障 2"=w557, "一级故障 3"=w558, "加热控制参数"=w559, "充电控制参数"=w560, "高压参数"=w552, "电池信息"=w553) -> (w550:T4)
                                n374 = control-ref of="二维码信息"() -> (w549:refnum<vi>)
                                n375 = local write "主板数据"(w550) -> ()
                                }
                                frame #1 {
                                n376 = control-ref of="主板数据"() -> (w561:refnum<vi>)
                                }
                                }
                                }
                                frame "从板" {
                                n377 = stacked-sequence {
                                tunnel: [_ w573] -> w562
                                frame #0 {
                                n378 = control-ref of="从板号"() -> (w567:refnum<vi>)
                                n379 = control-ref of="项目信息 2"() -> (w568:refnum<vi>)
                                n380 = control-ref of="电池组信息"() -> (w566:refnum<vi>)
                                n381 = control-ref of="加热控制参数"() -> (w569:refnum<vi>)
                                n382 = control-ref of="一级故障(从板)"() -> (w570:refnum<vi>)
                                n383 = control-ref of="二级故障(从板)"() -> (w571:refnum<vi>)
                                n384 = control-ref of="三级故障(从板)"() -> (w572:refnum<vi>)
                                n385 = control-ref of="均衡参数"() -> (w565:refnum<vi>)
                                n386 = local read "从板信息"() -> (w564:T2)
                                n387 = Bundle(cluster=w564, "从板号"=w567, "项目信息 2"=w568, "加热控制参数"=w569, "一级故障(从板)"=w570, "二级故障(从板)"=w571, "三级故障(从板)"=w572, "电池组信息(从板)"=w566, "均衡参数"=w565) -> (w563:T2)
                                n388 = local write "从板信息"(w563) -> ()
                                }
                                frame #1 {
                                n389 = control-ref of="从板信息"() -> (w573:refnum<vi>)
                                }
                                }
                                }
                              }
                              n390 = control-ref of="二维码信息 2"() -> (w536:refnum<vi>)
                              n391 = control-ref of="结果"() -> (w543:refnum<vi>)
                              n392 = control-ref of="从板个数"() -> (w539:refnum<vi>)
                              n393 = call "输出数据解析.vi"("主板引用"=w541, "从板引用"=w540, "板选择"=w538, "二维码信息"=w537, "错误代码"=w546, "命令序号"=w545, "输入数组"=w544, "命令"=w542, "进度引用"=w543, "从板个数"=w539, "从板二维码信息"=w536) -> ()  [unwired: 5 out]
                            }
                            frame True {
                              n394 = Index Array(array=w574, index #1=0 ("索引"), index #2=1 ("索引")) -> (element #1=w577:u8, element #2=w578:u8)
                              n395 = Join Numbers(hi=w577, lo=w578) -> ((hi.lo)=w576:u16)
                              n396 = Number To Hexadecimal String(2:w576) -> (0:w575:string)  [unwired: 1 out]
                              n397 = control-ref of="结果"() -> (w583:refnum<vi>)
                              n398 = Concatenate Strings("0x" ("字符串"), w575) -> (w584:string)
                              n399 = Build Array(w584) -> (w585:string[])
                              n400 = call "表格编辑.vi"("新元素/子数组"=w585, "活动单元格:单元格背景色"=u32 16740749, "MCListbox引用句柄"=w583) -> ()  [unwired: 9 out]
                            }
                          }
                          n401 = global write "EV05全局变量1.vi" "流控帧 2"(FALSE ("流控帧 2")) -> ()
                          n402 = global write "EV05全局变量1.vi" "输出数组"(i32[] []) -> ()
                          n403 = local write "控制1"(FALSE ("控制1")) -> ()
                          n404 = local write "消除"(FALSE ("消除")) -> ()
                        }
                      }
                    }
                    frame True {
                      # "写参数判定"
                      n405 = And(x="控制1", y=w591) -> (x .and. y?=w588:bool)
                      n406 = case shown="真" w588 {
                        tunnel: w590 -> [_ w598]
                        tunnel: w589 -> [_ w595]
                        frame False {
                        }
                        frame True {
                          n407 = call <vilib>:"Unset Busy.vi"() -> ()  [unwired: 2 in, 10 out]
                          n408 = case shown="\"主板\", 默认" w595 {
                            tunnel: [w599 w600] -> w597
                            frame "主板", Default {
                              n409 = local read "主板选项"() -> (w599:string)
                            }
                            frame "从板" {
                              n410 = local read "从板选项"() -> (w600:string)
                            }
                          }
                          n411 = control-ref of="结果"() -> (w596:refnum<vi>)
                          n412 = call "输入数据判定.vi"("主从选择"=w595, "主板选项"=w597, "进度引用"=w596, "错误代码"=w598) -> ()  [unwired: 2 in, 6 out]
                          n413 = global write "EV05全局变量1.vi" "流控帧 2"(FALSE ("流控帧 2")) -> ()
                          n414 = local write "控制1"(FALSE ("控制1")) -> ()
                          n415 = local write "消除"(FALSE ("消除")) -> ()
                        }
                      }
                      n416 = global write "EV05全局变量1.vi" "输出数组"(i32[] []) -> ()
                    }
                  }
                }
                frame "版本读取" {
                  n417 = local read "命令序号"() -> (w601:u8)
                  n418 = local read "从板板号"() -> (w604:u8)
                  n419 = local read "控制1"() -> (w605:bool)
                  n420 = call "多帧接收机制(EV05).vi"("can卡类型"=w612, "设备索引号"=w611, "CAN端口"=w610, "VCI_Receive"=w609, "命令"=w608, "板号"=w604, "命令序号"=w601) -> ("错误信号"=w602:bool, "输出数组"=w613:u8[], "读错误代码"=w603:u8[], "结束信号"=w607:bool)  [unwired: 1 in, 8 out]
                  n421 = And(x=w605, y=w607) -> (x .and. y?=w606:bool)
                  n422 = case shown="真" w606 {
                    tunnel: w613 -> [_ w621]
                    tunnel: w601 -> [_ w620]
                    tunnel: w608 -> [_ w619]
                    tunnel: w603 -> [_ w615]
                    tunnel: w602 -> [_ w614]
                    frame False {
                    }
                    frame True {
                      n423 = case shown="假" w614 {
                        tunnel: w621 -> [w625 _]
                        tunnel: w620 -> [w624 _]
                        tunnel: w619 -> [w623 _]
                        tunnel: w615 -> [w622 w849]
                        frame False {
                          n424 = case shown="89" w623 {
                            tunnel: w624 -> [_ w628]
                            tunnel: w625 -> [_ w627]
                            tunnel: w622 -> [_ _]
                            frame 0, Default {
                            }
                            frame 137 {
                              n425 = case shown="1" w628 {
                                tunnel: w627 -> [_ w656 w700 w720 w847]
                                frame 0, Default {
                                }
                                frame 1 {
                                w638 = "." ("字符串")
                                n426 = Array Subset(array=w656, index=0 ("索引"), length=14 ("长度")) -> (w669:u8[])
                                n427 = Index Array(array=w656, index=14 ("索引")) -> (element=w659:u8)
                                n428 = Index Array(array=w656, index #1=15 ("索引"), index #2=16 ("索引")) -> (element #1=w665:u8, element #2=w666:u8)
                                n429 = Index Array(array=w656, index #1=17 ("索引"), index #2=18 ("索引")) -> (element #1=w660:u8, element #2=w661:u8)
                                n430 = call "数组去零.vi"("输入"=w669) -> ("输出"=w644:dbl[])
                                n431 = Join Numbers(hi=w660, lo=w661) -> ((hi.lo)=w657:u16)
                                n432 = Join Numbers(hi=w665, lo=w666) -> ((hi.lo)=w658:u16)
                                n433 = Number To Decimal String(number=w659) -> (decimal integer string=w651:string)  [unwired: 1 out]
                                n434 = Byte Array To String(unsigned byte array=w644) -> (string=w643:string)
                                n435 = Number To Decimal String(number=w657) -> (decimal integer string=w639:string)  [unwired: 1 out]
                                n436 = Number To Decimal String(number=w658) -> (decimal integer string=w650:string)  [unwired: 1 out]
                                n437 = Array Subset(array=w656, index=21 ("索引"), length=7 ("长度")) -> (w653:u8[])
                                n438 = Concatenate Strings("V" ("字符串"), w651, w638, w650, w638, w639) -> (w648:string)
                                n439 = call "数组去零.vi"("输入"=w653) -> ("输出"=w636:dbl[])
                                n440 = Byte Array To String(unsigned byte array=w636) -> (string=w634:string)
                                n441 = call <vilib>:"Space Constant.vi"() -> ("String"=w635:string)
                                n442 = Equal?(x=w634, y=w635) -> (x = y?=w640:bool)
                                n443 = Concatenate Strings("-" ("字符串"), w634) -> (w641:string)
                                n444 = Select(t=w635, s=w640, f=w641) -> (s? t:f=w637:string)
                                n445 = Concatenate Strings(w643, "-" ("字符串"), w648, w637) -> (w630:string)
                                n446 = local read "项目软件版本"() -> (w632:string[])
                                n447 = local read "从板板号"() -> (w629:u8)
                                n448 = local write "项目软件版本号"(w630) -> ()
                                n449 = Replace Array Subset(array=w632, new element=w630, index=w629) -> (w631:string[])
                                n450 = control-ref of="结果"() -> (w647:refnum<vi>)
                                n451 = local write "项目软件版本"(w631) -> ()
                                n452 = Build Array("项目软件版本     读取完成" ("读取结果")) -> (w645:string[])
                                n453 = call "表格编辑(版本读取).vi"("新元素/子数组"=w645, "活动单元格:单元格背景色"=u32 6618880, "MCListbox引用句柄"=w647) -> ()  [unwired: 9 out]
                                }
                                frame 2 {
                                w683 = ""
                                w680 = "." ("字符串")
                                n454 = Array Subset(array=w700, index=0 ("索引"), length=14 ("长度")) -> (w688:u8[])
                                n455 = Index Array(array=w700, index=14 ("索引")) -> (element=w703:u8)
                                n456 = Index Array(array=w700, index #1=15 ("索引"), index #2=16 ("索引")) -> (element #1=w709:u8, element #2=w710:u8)
                                n457 = Index Array(array=w700, index #1=17 ("索引"), index #2=18 ("索引")) -> (element #1=w704:u8, element #2=w705:u8)
                                n458 = Join Numbers(hi=w704, lo=w705) -> ((hi.lo)=w701:u16)
                                n459 = Join Numbers(hi=w709, lo=w710) -> ((hi.lo)=w702:u16)
                                n460 = Number To Decimal String(number=w701) -> (decimal integer string=w681:string)  [unwired: 1 out]
                                n461 = call "数组去零.vi"("输入"=w688) -> ("输出"=w687:dbl[])
                                n462 = Number To Decimal String(number=w703) -> (decimal integer string=w695:string)  [unwired: 1 out]
                                n463 = Number To Decimal String(number=w702) -> (decimal integer string=w694:string)  [unwired: 1 out]
                                n464 = Array Subset(array=w700, index=21 ("索引"), length=7 ("长度")) -> (w697:u8[])
                                n465 = Byte Array To String(unsigned byte array=w687) -> (string=w682:string)
                                n466 = call "数组去零.vi"("输入"=w697) -> ("输出"=w679:dbl[])
                                n467 = Concatenate Strings("V" ("字符串"), w695, w680, w694, w680, w681) -> (w692:string)
                                n468 = Byte Array To String(unsigned byte array=w679) -> (string=w677:string)
                                n469 = Equal?(x=w683, y=w677) -> (x = y?=w684:bool)
                                n470 = Concatenate Strings("-" ("字符串"), w677) -> (w685:string)
                                n471 = Select(t=w683, s=w684, f=w685) -> (s? t:f=w678:string)
                                n472 = Concatenate Strings(w682, "-" ("字符串"), w692, w678) -> (w673:string)
                                n473 = local read "平台软件版本"() -> (w675:string[])
                                n474 = local read "从板板号"() -> (w672:u8)
                                n475 = local write "平台软件版本号"(w673) -> ()
                                n476 = Replace Array Subset(array=w675, new element=w673, index=w672) -> (w674:string[])
                                n477 = control-ref of="结果"() -> (w690:refnum<vi>)
                                n478 = local write "平台软件版本"(w674) -> ()
                                n479 = Build Array("平台软件版本     读取完成" ("读取结果")) -> (w689:string[])
